vi "PIL_Main.vi"() -> ()   [LabVIEW 2024]
uses:
  controls/EXPERIMENT_Inputs.ctl
  controls/LASER_Inputs.ctl
  controls/LAMP_Inputs.ctl
  controls/GAS_Inputs.ctl
  controls/EXPERT_Inputs.ctl
  controls/XML_Inputs.ctl
  controls/SOFTWARE_Inputs.ctl
  controls/HSDIO_6541_Inputs.ctl
  <instrlib>/niHSDIO/niHSDIO.llb/niHSDIO_ctl Trigger Source Values (Ring).ctl
  controls/AWG_5421_Inputs.ctl
  <instrlib>/niFgen/niFgen.llb/niFgen_ctl Trigger Source Values (Ring).ctl
  controls/DIGIT_5122_Inputs.ctl
  <instrlib>/niScope/Controls/niScope trigger source.ctl
  controls/AO_6711_Inputs.ctl
  controls/AO_6738_Inputs.ctl
  controls/VOLTAGES_Inputs.ctl
  controls/HEXA_Inputs.ctl
  controls/QUAD_Inputs.ctl
  controls/SEQUENCE_Inputs.ctl
  controls/EXCIT_Inputs.ctl
  controls/DATA_Inputs.ctl
  controls/TIMING_Inputs.ctl
  controls/PROCESSING_Inputs.ctl
  controls/TRAPPING_Inputs.ctl
  controls/RF_TRAPPING_Inputs.ctl
  controls/SPECTRUM.ctl
  controls/EXCIT_Table.ctl
  controls/TIMING_Table.ctl
  controls/TIMING_Mandatory_Items.ctl
  controls/TIMING_Optional_Items.ctl
  controls/PIL_Status.ctl
  controls/LOOPS_Inputs.ctl
  controls/OPO_Inputs.ctl
  controls/QMH_UI_Cluster.ctl
  controls/QMH_UI_References.ctl
  controls/QMH_UI_Report.ctl
  controls/QMH_UI_Command.ctl
  controls/QMH_ICR_Command.ctl
  controls/QMH_Status.ctl
  controls/EXPERT_Path_Selector.ctl
  <vilib>/Utility/error.llb/DialogType.ctl
  Global_Variables.vi
panel:
  in  "Save As":bool
  in  "error in (no error)":errorcluster
  in  "Start":bool
  in  "Load":bool
  in  "Exit":bool
  in  "Tabs":T1(tab)=enum."Sequence"
  out "SPECTRUM":T2={"Day Path"=path "D:/PIRENEA/DATA/2016/data_2016_01_01", "Spectrum Name"="2016_01_01_000.A00", "Accumulated"=FALSE, "Stored in Database"=FALSE, "From a Set of"=0, "Quality Flag"="Optimal"}
  in  "Change Experiment":bool
  out "EXPERIMENT Inputs":T3={"Setup"="", "Date"="", "User Name"="", "Comment"="", "Experiment Procedures"=[], "Chemical Source"="", "Sample Components"=[], "Species"=[], "Laser 1"={"Used"=TRUE, "Name"="Spectroscopy", "Wavelength"=1000.0, "Energy"=25.0}, "Laser 2"={"Used"=TRUE, "Name"="Spectroscopy", "Wavelength"=1000.0, "Energy"=25.0}, "Laser 3"={"Used"=TRUE, "Name"="Spectroscopy", "Wavelength"=1000.0, "Energy"=25.0}, "Laser 4"={"Used"=TRUE, "Name"="Spectroscopy", "Wavelength"=1000.0, "Energy"=25.0}, "Laser 5"={"Used"=TRUE, "Name"="Spectroscopy", "Wavelength"=1000.0, "Energy"=25.0}, "Lamp 1"={"Used"=TRUE, "Name"="Spectroscopy", "Wavelength"=1000.0, "Attenuation"=25.0}, "Lamp 2"={"Used"=TRUE, "Name"="Spectroscopy", "Wavelength"=1000.0, "Attenuation"=25.0}, "Gas 1"={"Used"=TRUE, "Name"="Spectroscopy", "Pressure"=1000.0}, "Gas 2"={"Used"=TRUE, "Name"="Spectroscopy", "Pressure"=1000.0}, "Gas 3"={"Used"=TRUE, "Name"="Spectroscopy", "Pressure"=1000.0}, "Gas 4"={"Used"=TRUE, "Name"="Spectroscopy", "Pressure"=1000.0}, "Gas 5"={"Used"=TRUE, "Name"="Spectroscopy", "Pressure"=1000.0}} caption="EXCIT Paths"
  in  "Change Voltages":bool
  out "VOLTAGES Inputs":T7={"Hexa 1"={"Used"=FALSE, "Voltage"=0.0}, "Hexa 2"={"Used"=FALSE, "Voltage"=0.0}, "Hexa 3"={"Used"=FALSE, "Voltage"=0.0}, "Quad 1"={"Used"=TRUE, "Voltage"=25.0}, "Quad 2"={"Used"=TRUE, "Voltage"=25.0}, "Quad 3"={"Used"=TRUE, "Voltage"=25.0}}
  out "SEQUENCE Inputs":T10={"EXCIT Inputs"={"Number of Excitations"=1, "Script Text"="script  excit1wfm\r    wait until scriptTrigger0\r    generate Sinus250to500a25dur1200fs10\rend script", "Table of Waveforms"=["Sinus250to500a25dur1200fs10"]}, "DATA Inputs"={"Record Length"=524000, "Sample Rate"=2000000.0, "Data Type"=0, "Vertical Range"=2.0, "Acquisition Duration"=100000.0}, "TIMING Inputs"={"Number of Acquisitions "=1, "Number of Accumulations"=1, "Table of Waveforms"=["", "", "", "", "", "", "", "", "", "", "", ""], "Script Text"=""}, "PROCESSING Inputs"={"Reference Mass"=300.0939, "Cyclotron Freq"=255.727, "Magnetron Freq"=0.001}, "TRAPPING Inputs"={"Number of Channels"=4, "Init Values"=[2.0, 9.0, 9.0, 2.0], "Opening Values"=[0.0, 0.0, 0.0, 0.0], "Trapping Values"=[2.0, 9.0, 9.0, 2.0], "Emptying Values"=[-10.0, -10.0, -10.0, -10.0], "Adiabatic ON"=FALSE, "Adiabatic Duration"=0, "Adiabatic Waveforms"=["Adiabatic_None_2_2_2000", "Adiabatic_Ramp_9_0_2000", "Adiabatic_DoubleRamp_9_0_2000", "Adiabatic_RC_2_0_2000.bin"], "Ions Refill ON"=FALSE, "Number of Ions Refills"=4}, "RF_TRAPPING Inputs"={"Init Values"=[0.0, 1.0, 1.0, 0.0], "Opening Values"=[0.0, -4.0, 1.0, 0.0], "Trapping Values"=[0.0, 1.0, 1.0, 0.0], "Emptying Values"=[0.0, 1.0, -7.0, 0.0], "RF Trap ON"=FALSE, "RF Accums"=1, "Number of Voltages"=4}} {"RF_TRAPPING Inputs"."RF Accums" min=1 max=100; "RF_TRAPPING Inputs"."Trapping Values" min=-10.0 max=10.0; "RF_TRAPPING Inputs"."Init Values" min=-10.0 max=10.0; "RF_TRAPPING Inputs"."Emptying Values" min=-10.0 max=10.0; "RF_TRAPPING Inputs"."Opening Values" min=-10.0 max=10.0; "TRAPPING Inputs"."Number of Ions Refills" min=1 max=1000; "TRAPPING Inputs"."Trapping Values" min=-10.0 max=10.0; "TRAPPING Inputs"."Init Values" min=-10.0 max=10.0; "TRAPPING Inputs"."Emptying Values" min=-10.0 max=10.0; "TRAPPING Inputs"."Opening Values" min=-10.0 max=10.0; "PROCESSING Inputs"."Magnetron Freq" format="%.5g"; "PROCESSING Inputs"."Cyclotron Freq" format="%.5g"; "PROCESSING Inputs"."Reference Mass" format="%.5g"; "TIMING Inputs"."Number of Accumulations" min=0 max=50 step=1; "TIMING Inputs"."Number of Acquisitions" min=1 max=10 step=1; "DATA Inputs"."Vertical Range" items=["0.2"=0.2, "0.4"=0.4, "1"=1.0, "2"=2.0, "4"=4.0, "10"=10.0]; "DATA Inputs"."Data Type" items=["I16", "DBL"]; "DATA Inputs"."Sample Rate" items=["1 MHz"=1000000.0, "2 MHz"=2000000.0, "5 MHz"=5000000.0, "10 MHz"=10000000.0, "20 MHz"=20000000.0, "25 MHz"=25000000.0, "50 MHz"=50000000.0, "100 MHz"=100000000.0]; "EXCIT Inputs"."Number of Excitations" min=1 max=10}
  in  "Change Sequence":bool
  in  "Change Expert":bool
  out "EXPERT Inputs":T17={"XML Inputs"={"Version Tag Name"="XML_Version", "Version String"="1.1"}, "SOFTWARE Inputs"={"Application Directory"=path "D:/S.O.F.T.S/LABVIEW/PIL", "Software Version"="17.0f2", "Data Path"=path "D:/PIRENEA/DATA", "XML Path"=path "D:/PIRENEA/DATA", "XML File Filter"="*.xml", "XML Saved Path"=path "D:/PIRENEA/SAVED_XML", "Excit Scripts Path"=path "D:/PIRENEA/TECHNICAL/EXCIT_SCRIPTS", "Excit Scripts File Filter"="*.txt", "Excit Waveforms Path"=path "D:/PIRENEA/TECHNICAL/EXCIT_WFMS", "Excit Waveforms File Filter"="*.bin", "Timing Scripts Path"=path "D:/PIRENEA/TECHNICAL/TIMING_SCRIPTS", "Timing Scripts File Filter"="*.txt", "Timing Waveforms Path"=path "D:/PIRENEA/TECHNICAL/TIMING_WFMS", "Timing Waveforms File Filter"="*.bin", "Trapping Waveforms Path"=path "D:/PIRENEA/TECHNICAL/TRAPPING_WFMS", "Trapping Waveforms File Filter"="*.bin"}, "HSDIO 6541 Inputs"={"Resource Name"="HSDIO_6541", "Clock Rate"=1000000.0, "Trigger Source"="PFI0"}, "AWG 5421 Inputs"={"Resource Name"="AWG_5421", "Sample Rate"=10000000.0, "Trigger Type"=2, "Trigger Source"="PFI0", "Waveform Gain"=0.31, "Digital Filter ON"=TRUE}, "DIGIT 5122 Inputs"={"Sample Rate"=5000000.0, "Resource Name"="DIGIT_5122", "Channel Name"="0", "Trigger Source"="VAL_EXTERNAL", "Vertical Range"=2.0, "Trigger Level"=3.0}, "AO 6711 Inputs"={"Physical Channels"="AO_6711/ao0:3", "Min Voltage"=-10.0, "Max Voltage"=10.0, "Trigger Source"="/AO_6711/PFI3", "Counter"="AO_6711/ctr0"}, "AO 6738 Inputs"={"Physical Channels"="AO_6738/ao0:3", "Min Voltage"=-10.0, "Max Voltage"=10.0, "Trigger Source"="/AO_6738/PFI2", "Counter"="AO_6738/ctr0"}} {"AO 6738 Inputs"."Max Voltage" min=-10.0 max=10.0; "AO 6738 Inputs"."Min Voltage" min=-10.0 max=10.0; "AWG 5421 Inputs"."Sample Rate" format="%.2p"; "AWG 5421 Inputs"."Trigger Type" items=["None", "Software Edge", "Digital Edge", "Digital Level"]; "AO 6711 Inputs"."Max Voltage" min=-10.0 max=10.0; "AO 6711 Inputs"."Min Voltage" min=-10.0 max=10.0; "HSDIO 6541 Inputs"."Clock Rate" format="%.2p"; "DIGIT 5122 Inputs"."Trigger Level" format="%.2f"; "DIGIT 5122 Inputs"."Vertical Range" format="%.2f"; "DIGIT 5122 Inputs"."Sample Rate" step=65535.0 format="%#_3p"}
  in  "LOOPS Inputs":T28={"Number of Loops"=0, "Loop Current Value"=0, "OPO Inputs"={"OPO AutoAlignment ON"=FALSE, "OPO Start Value"=210.0, "OPO Stop Value"=270.0, "OPO Step"=30.0}} {"OPO Inputs"."OPO Step" min=0.5 max=60.0 format="%#.1f"; "OPO Inputs"."OPO Stop Value" min=210.0 max=270.0 format="%#.1f"; "OPO Inputs"."OPO Start Value" min=210.0 max=270.0 format="%#.1f"}
  in  "Change Loops":bool
  in  "Excit Test":bool caption="AWG5421 Board"
  out "TIMING Script":string
  in  "Change Scientist":bool
  out "TIMING Table":T30={"Mandatory Items"={"Script Name"="", "GINI Time Period"=100.0, "HSDIO Delay"=60.0, "Shutter Duration before"=50.0, "Shutter Duration after"=50.0, "Filter Tau"=2.0, "Trapping Delay"=600.0, "Trapping Duration"=300.0, "Emtyping Duration"=1000.0}, "Optional Items"={"Eject"=0, "Acq"=0, "Excit"=0, "Gas"=0, "Laser"=0, "Lamp"=0}, "Times Table"=[["Excit1", "name", "Swift", "0.5", "1200", "70", "150", "550", "0", "0", "0"]]} {"Optional Items"."Laser" min=0 max=3; "Optional Items"."Gas" min=0 max=5; "Mandatory Items"."GINI Time Period" min=100000.0 max=1000000.0 format="%#_7g"; "Mandatory Items"."Shutter Duration after" min=2.0 max=100000.0; "Mandatory Items"."HSDIO Delay" min=60.0 max=100.0; "Mandatory Items"."Shutter Duration before" min=2.0 max=100000.0; "Mandatory Items"."Filter Tau" min=1000.0 max=2000.0; "Mandatory Items"."Trapping Delay" min=2.0; "Mandatory Items"."Emtyping Duration" min=2.0 format="%#_8g"; "Mandatory Items"."Trapping Duration" min=2.0}
  out "EXCIT Table":T33={"Number of Excits"=0, "Number of Ejects"=0, "Sampling Frequency"=0.0, "Waveforms Table"=[["Excit1", "name", "Swift", "0.5", "1200", "70", "150", "550", "0", "0", "0"]]}
  out "PIL Status":T34
  # "Lasers"
  # "nm"
  # "mJ"
  # "Lamps"
  # "nm"
  # "dB"
  # "Gas"
  # "bar"
  # "HEXAPOLE"
  # "QUADRIPOLE"
  # "RF_V1"
  # "RF_V2"
  # "RF_V3"
  # "RF_V4"
  # "GO_out"
  # "Gout"
  # "GI_in"
  # "Gin"
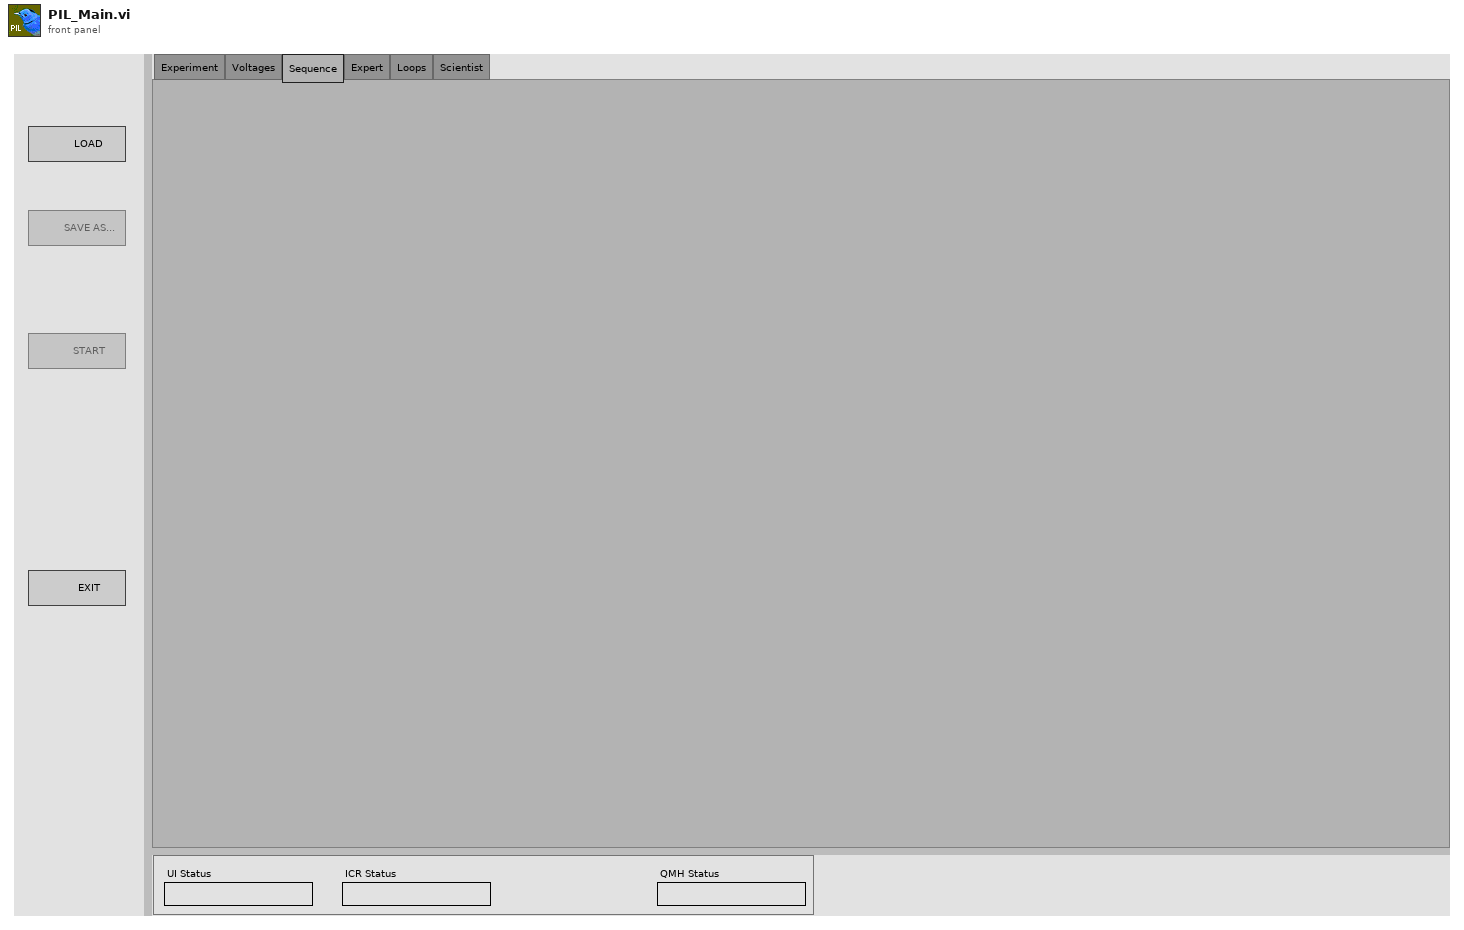
[diagram p1: front panel]
types:
  T1 = enum32{"Experiment", "Voltages", "Sequence", "Expert", "Loops", "Scientist"}
  T2 = typedef "SPECTRUM.ctl" = cluster{"Day Path":path, "Spectrum Name":string, "Accumulated":bool, "Stored in Database":bool, "From a Set of":i16, "Quality Flag":string}
  T3 = typedef "EXPERIMENT_Inputs.ctl" = cluster{"Setup":string, "Date":string, "User Name":string, "Comment":string, "Experiment Procedures":string[], "Chemical Source":string, "Sample Components":string[], "Species":string[], "Laser 1":T4, "Laser 2":T4, "Laser 3":T4, "Laser 4":T4, "Laser 5":T4, "Lamp 1":T5, "Lamp 2":T5, "Gas 1":T6, "Gas 2":T6, "Gas 3":T6, "Gas 4":T6, "Gas 5":T6}
  T4 = typedef "LASER_Inputs.ctl" = cluster{"Used":bool, "Name":string, "Wavelength":dbl, "Energy":dbl}
  T5 = typedef "LAMP_Inputs.ctl" = cluster{"Used":bool, "Name":string, "Wavelength":dbl, "Attenuation":dbl}
  T6 = typedef "GAS_Inputs.ctl" = cluster{"Used":bool, "Name":string, "Pressure":dbl}
  T7 = typedef "VOLTAGES_Inputs.ctl" = cluster{"Hexa 1":T8, "Hexa 2":T8, "Hexa 3":T8, "Quad 1":T9, "Quad 2":T9, "Quad 3":T9}
  T8 = typedef "HEXA_Inputs.ctl" = cluster{"Used":bool, "Voltage":dbl}
  T9 = typedef "QUAD_Inputs.ctl" = cluster{"Used":bool, "Voltage":dbl}
  T10 = typedef "SEQUENCE_Inputs.ctl" = cluster{"EXCIT Inputs":T11, "DATA Inputs":T12, "TIMING Inputs":T13, "PROCESSING Inputs":T14, "TRAPPING Inputs":T15, "RF_TRAPPING Inputs":T16}
  T11 = typedef "EXCIT_Inputs.ctl" = cluster{"Number of Excitations":i32, "Script Text":string, "Table of Waveforms":string[]}
  T12 = typedef "DATA_Inputs.ctl" = cluster{"Record Length":i32, "Sample Rate":dbl, "Data Type":u8, "Vertical Range":dbl, "Acquisition Duration":dbl}
  T13 = typedef "TIMING_Inputs.ctl" = cluster{"Number of Acquisitions ":i16, "Number of Accumulations":i16, "Table of Waveforms":string[], "Script Text":string}
  T14 = typedef "PROCESSING_Inputs.ctl" = cluster{"Reference Mass":dbl, "Cyclotron Freq":dbl, "Magnetron Freq":dbl}
  T15 = typedef "TRAPPING_Inputs.ctl" = cluster{"Number of Channels":i32, "Init Values":dbl[], "Opening Values":dbl[], "Trapping Values":dbl[], "Emptying Values":dbl[], "Adiabatic ON":bool, "Adiabatic Duration":i32, "Adiabatic Waveforms":string[], "Ions Refill ON":bool, "Number of Ions Refills":i32}
  T16 = typedef "RF_TRAPPING_Inputs.ctl" = cluster{"Init Values":dbl[], "Opening Values":dbl[], "Trapping Values":dbl[], "Emptying Values":dbl[], "RF Trap ON":bool, "RF Accums":i32, "Number of Voltages":i32}
  T17 = typedef "EXPERT_Inputs.ctl" = cluster{"XML Inputs":T18, "SOFTWARE Inputs":T19, "HSDIO 6541 Inputs":T20, "AWG 5421 Inputs":T22, "DIGIT 5122 Inputs":T24, "AO 6711 Inputs":T26, "AO 6738 Inputs":T27}
  T18 = typedef "XML_Inputs.ctl" = cluster{"Version Tag Name":string, "Version String":string}
  T19 = typedef "SOFTWARE_Inputs.ctl" = cluster{"Application Directory":path, "Software Version":string, "Data Path":path, "XML Path":path, "XML File Filter":string, "XML Saved Path":path, "Excit Scripts Path":path, "Excit Scripts File Filter":string, "Excit Waveforms Path":path, "Excit Waveforms File Filter":string, "Timing Scripts Path":path, "Timing Scripts File Filter":string, "Timing Waveforms Path":path, "Timing Waveforms File Filter":string, "Trapping Waveforms Path":path, "Trapping Waveforms File Filter":string}
  T20 = typedef "HSDIO_6541_Inputs.ctl" = cluster{"Resource Name":refnum<k15>, "Clock Rate":dbl, "Trigger Source":T21}
  T21 = typedef "niHSDIO_ctl Trigger Source Values (Ring).ctl" = string
  T22 = typedef "AWG_5421_Inputs.ctl" = cluster{"Resource Name":refnum<k15>, "Sample Rate":dbl, "Trigger Type":u16, "Trigger Source":T23, "Waveform Gain":dbl, "Digital Filter ON":bool}
  T23 = typedef "niFgen_ctl Trigger Source Values (Ring).ctl" = string
  T24 = typedef "DIGIT_5122_Inputs.ctl" = cluster{"Sample Rate":dbl, "Resource Name":refnum<k15>, "Channel Name":string, "Trigger Source":T25, "Vertical Range":dbl, "Trigger Level":dbl}
  T25 = typedef "niScope trigger source.ctl" = string
  T26 = typedef "AO_6711_Inputs.ctl" = cluster{"Physical Channels":tag, "Min Voltage":dbl, "Max Voltage":dbl, "Trigger Source":tag, "Counter":tag}
  T27 = typedef "AO_6738_Inputs.ctl" = cluster{"Physical Channels":tag, "Min Voltage":dbl, "Max Voltage":dbl, "Trigger Source":tag, "Counter":tag}
  T28 = typedef "LOOPS_Inputs.ctl" = cluster{"Number of Loops":i16, "Loop Current Value":i16, "OPO Inputs":T29}
  T29 = typedef "OPO_Inputs.ctl" = cluster{"OPO AutoAlignment ON":bool, "OPO Start Value":dbl, "OPO Stop Value":dbl, "OPO Step":dbl}
  T30 = typedef "TIMING_Table.ctl" = cluster{"Mandatory Items":T31, "Optional Items":T32, "Times Table":string[][]}
  T31 = typedef "TIMING_Mandatory_Items.ctl" = cluster{"Script Name":string, "GINI Time Period":dbl, "HSDIO Delay":dbl, "Shutter Duration before":dbl, "Shutter Duration after":dbl, "Filter Tau":dbl, "Trapping Delay":dbl, "Trapping Duration":dbl, "Emtyping Duration":dbl}
  T32 = typedef "TIMING_Optional_Items.ctl" = cluster{"Eject":u32, "Acq":i32, "Excit":u32, "Gas":i32, "Laser":i32, "Lamp":i32}
  T33 = typedef "EXCIT_Table.ctl" = cluster{"Number of Excits":u16, "Number of Ejects":u16, "Sampling Frequency":dbl, "Waveforms Table":string[][]}
  T34 = typedef "PIL_Status.ctl" = cluster{"UI Status":string, "ICR Status":string, "QMH Status":string}
  T35 = typedef "QMH_UI_Cluster.ctl" = cluster{"QMH UI References":T36, "QMH UI Report":T37}
  T36 = typedef "QMH_UI_References.ctl" = cluster{"Refnum Load":refnum<vi>, "Refnum Save As":refnum<vi>, "Refnum Start":refnum<vi>, "Refnum Exit":refnum<vi>, "Refnum Tabs":refnum<vi>, "Refnum SPECTRUM":refnum<vi>, "Refnum EXPERIMENT":refnum<vi>, "Refnum VOLTAGES":refnum<vi>, "Refnum SEQUENCE":refnum<vi>, "Refnum EXPERT":refnum<vi>, "Refnum LOOPS":refnum<vi>, "Refnum EXCIT Table":refnum<vi>, "Refnum TIMING Table":refnum<vi>, "Refnum CHANGE Experiment":refnum<vi>, "Refnum CHANGE Voltages":refnum<vi>, "Refnum CHANGE Sequence":refnum<vi>, "Refnum CHANGE Expert":refnum<vi>, "Refnum CHANGE Loops":refnum<vi>, "Refnum CHANGE Scientist":refnum<vi>, "Refnum PIL Status":refnum<vi>}
  T37 = typedef "QMH_UI_Report.ctl" = cluster{"UI Status":T38, "ICR Status":T39, "QMH Status":T40}
  T38 = typedef "QMH_UI_Command.ctl" = enum16{"Initialize", "UI Load", "UI Save", "UI Save As", "UI Change Experiment", "UI Change Voltages", "UI Change Sequence", "UI Change Expert", "UI Change Loops", "UI Change Scientist", "Ready to Start", "UI Start", "Waiting for ICR", "UI Exit", "Update Experiment", "Update Report", "Update ICR Status", "Waiting for User"}
  T39 = typedef "QMH_ICR_Command.ctl" = enum16{"Initialize", "Sequence Loop Setup", "Sequence Setup", "ICR Start", "ICR Stop", "Hardware Setup", "Next Sequence Loop", "Next Accumulation", "Waiting for Trigger", "Sequence Started", "Sequence Finished", "Sequence Loop Done", "Writing Data", "Hardware Reset", "Exit"}
  T40 = typedef "QMH_Status.ctl" = enum16{"Init", "Loading", "Setup", "Ready to Start", "Started", "Idle"}
  T41 = typedef "EXPERT_Path_Selector.ctl" = enum16{"Application", "Resources", "Data", "XML", "XML Saved", "Load Directory"}
  T42 = typedef "QMH_UI_Message.ctl" = cluster{"Command":T38, "Data":variant}
  T43 = typedef "DialogType.ctl" = u16
  T44 = enum32{"invalid app kind", "Development System", "Run Time System", "Student Edition", "Embedded LabVIEW", "Evaluation", "Custom"}
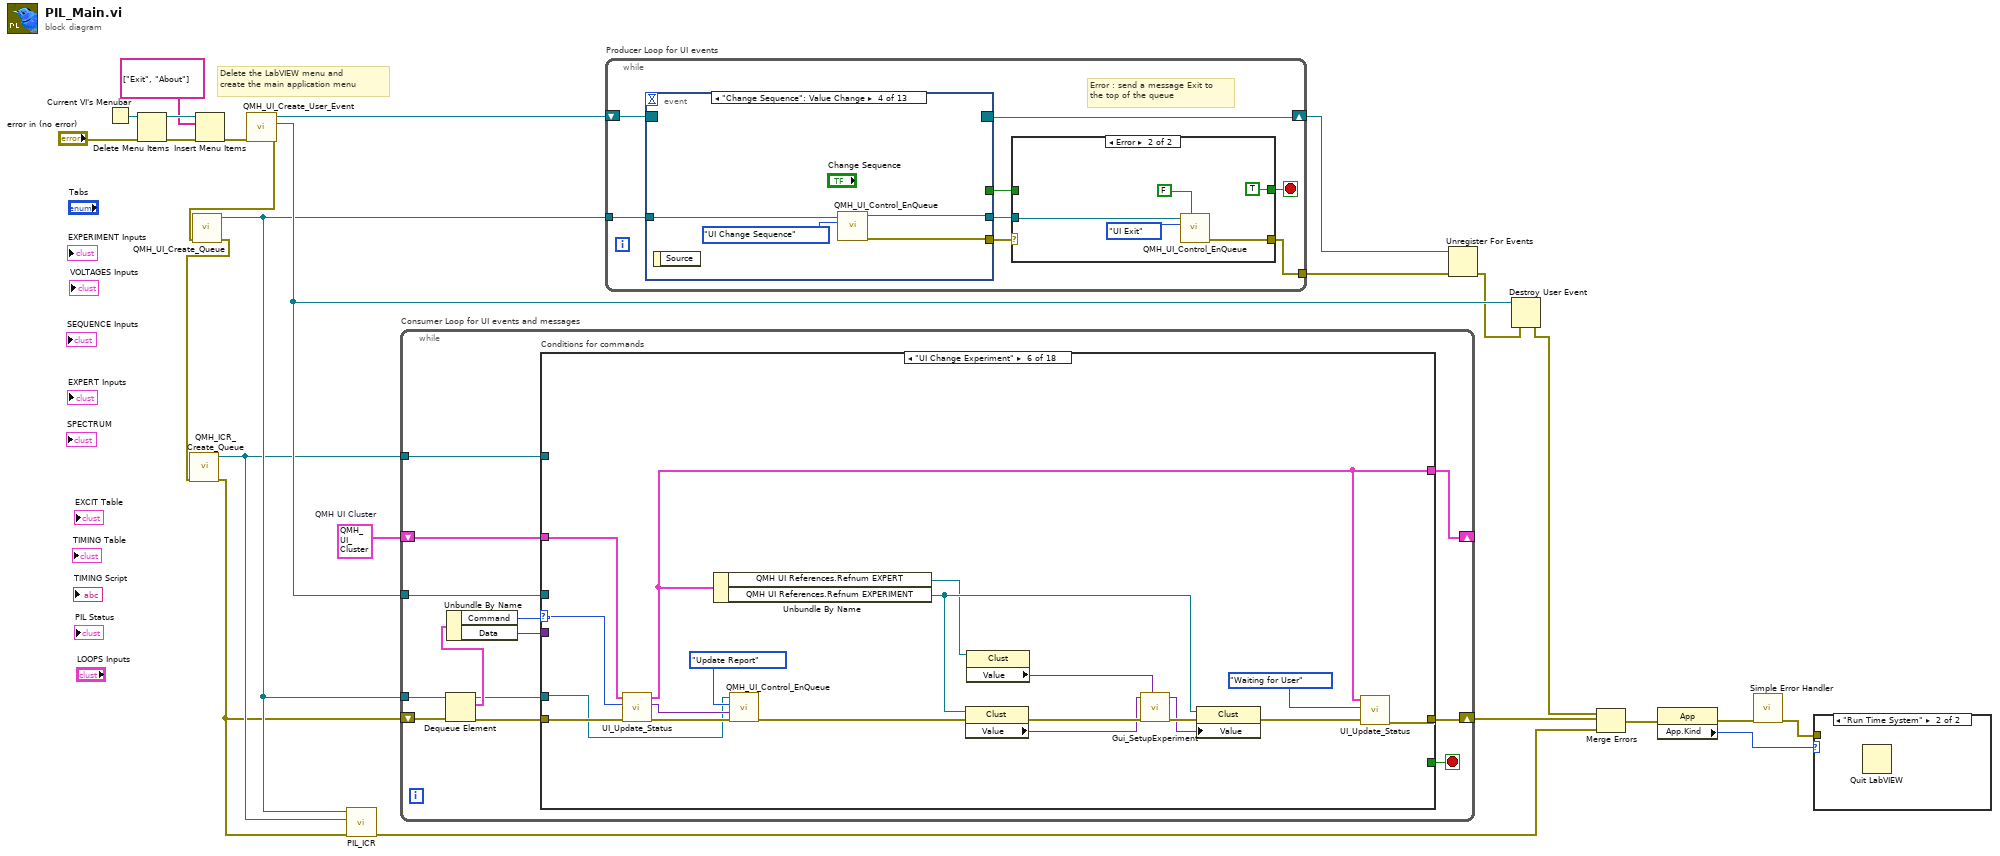
[diagram p0: block diagram]
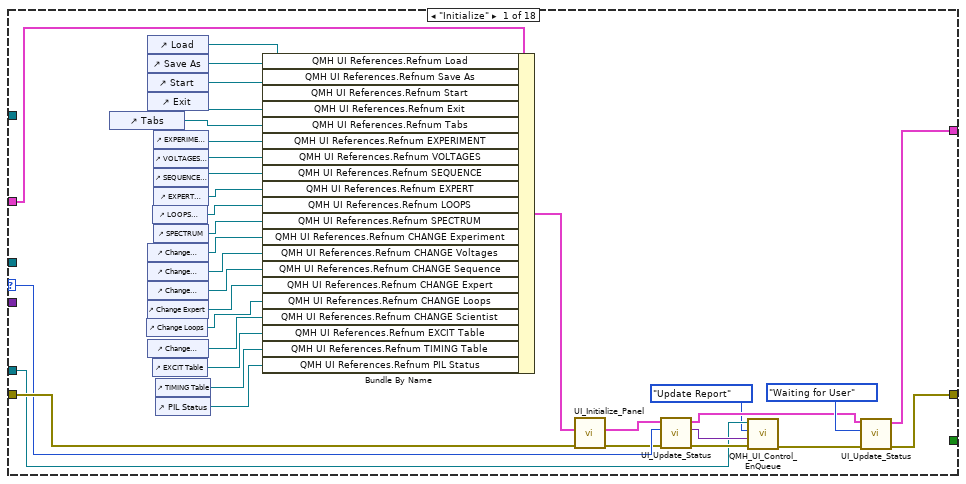
[diagram p2: hidden frame]
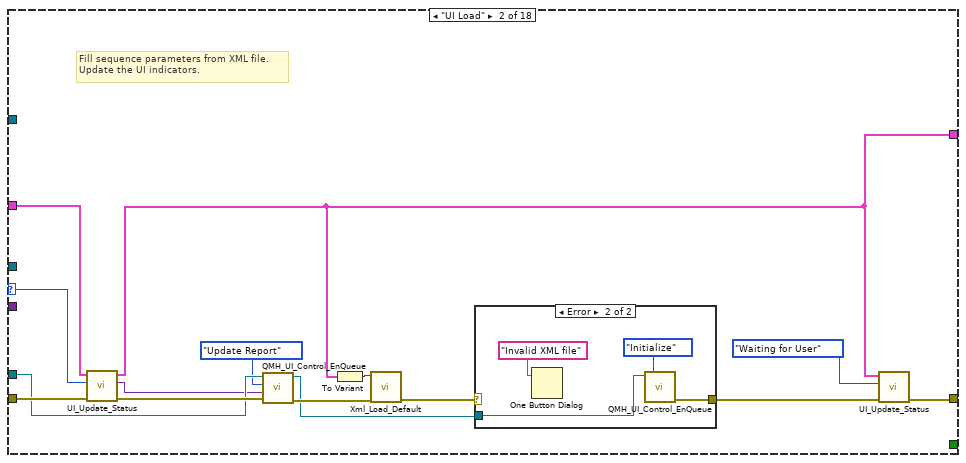
[diagram p3: hidden frame]
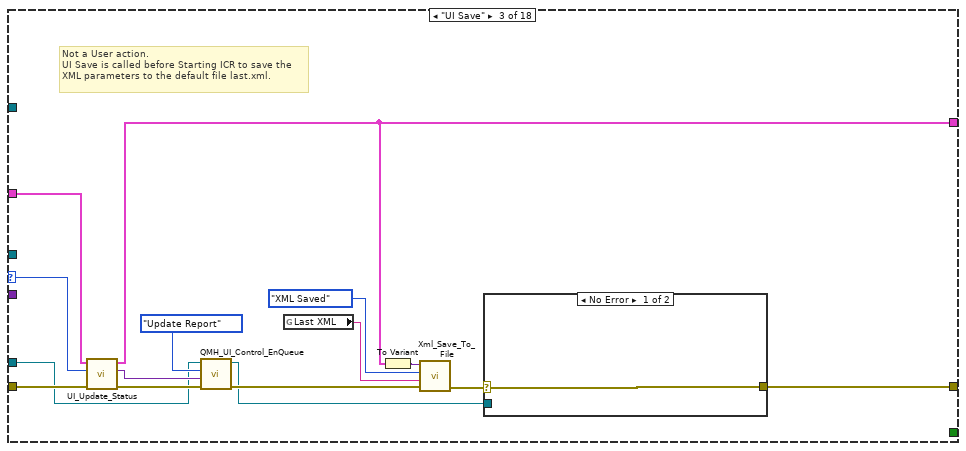
[diagram p5: hidden frame]
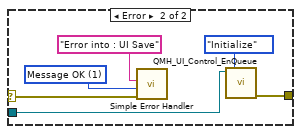
[diagram p6: hidden frame]
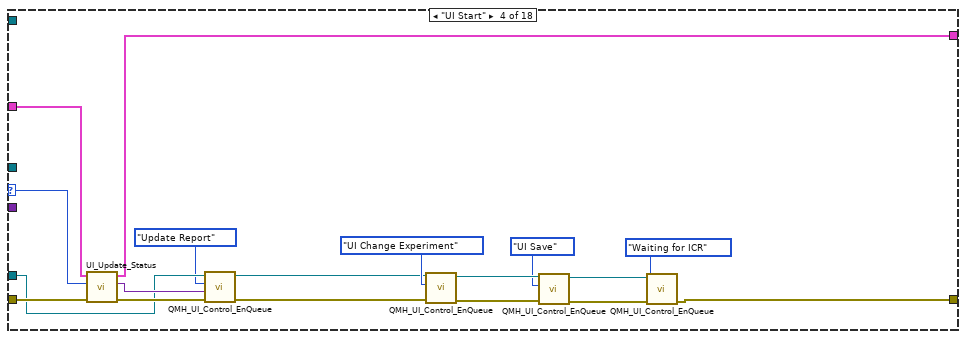
[diagram p7: hidden frame]
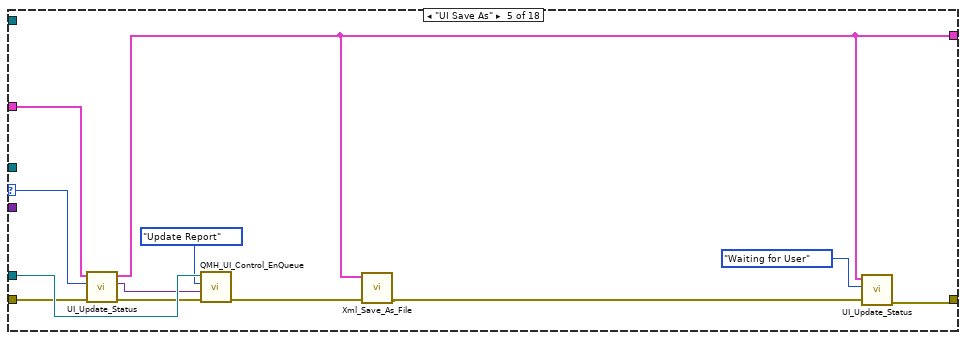
[diagram p8: hidden frame]
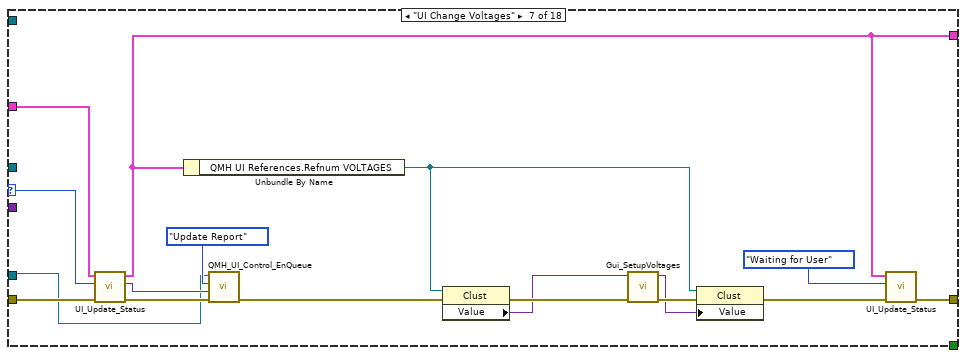
[diagram p9: hidden frame]
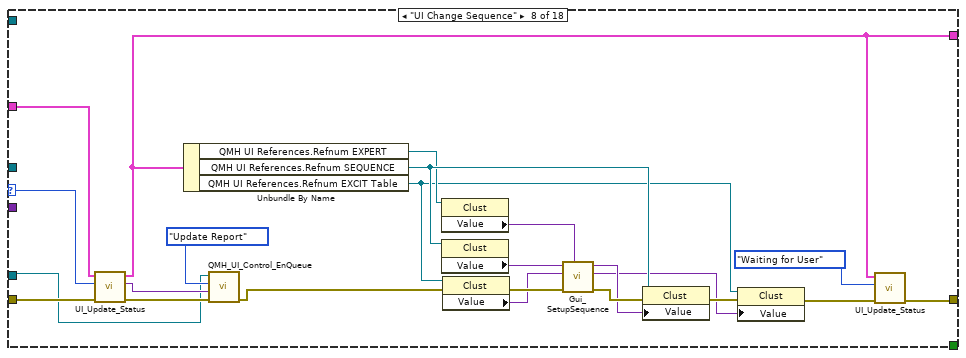
[diagram p10: hidden frame]
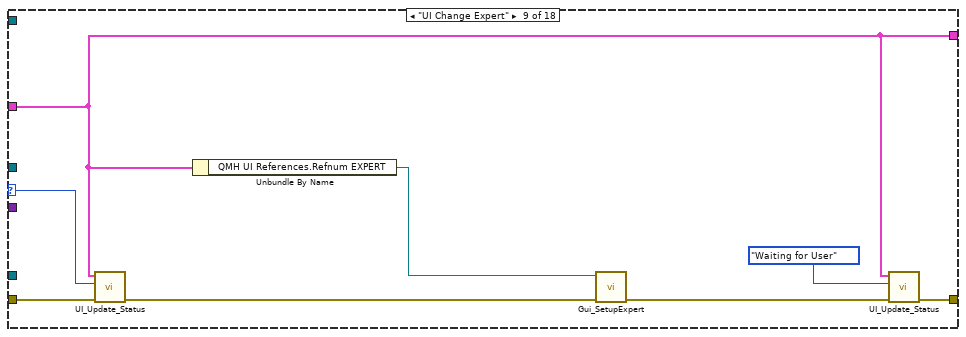
[diagram p11: hidden frame]
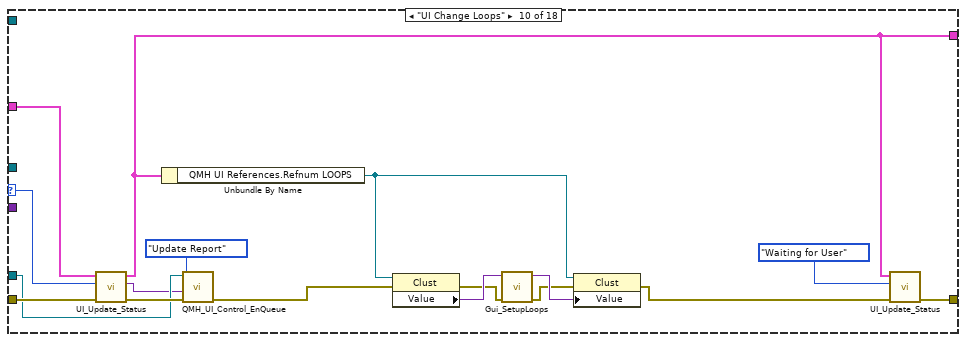
[diagram p12: hidden frame]
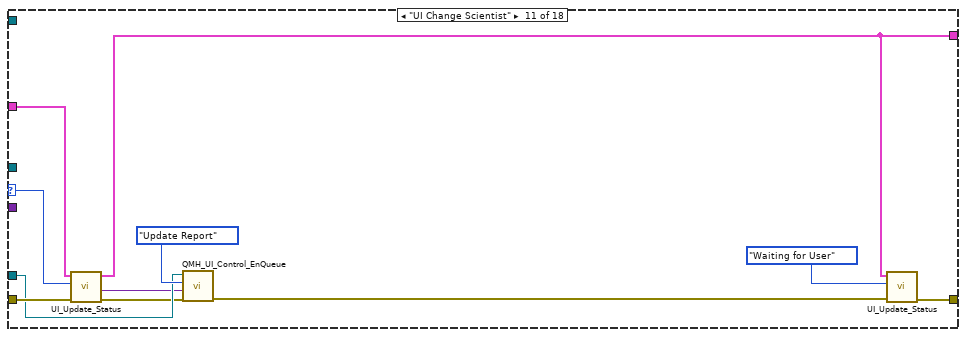
[diagram p13: hidden frame]
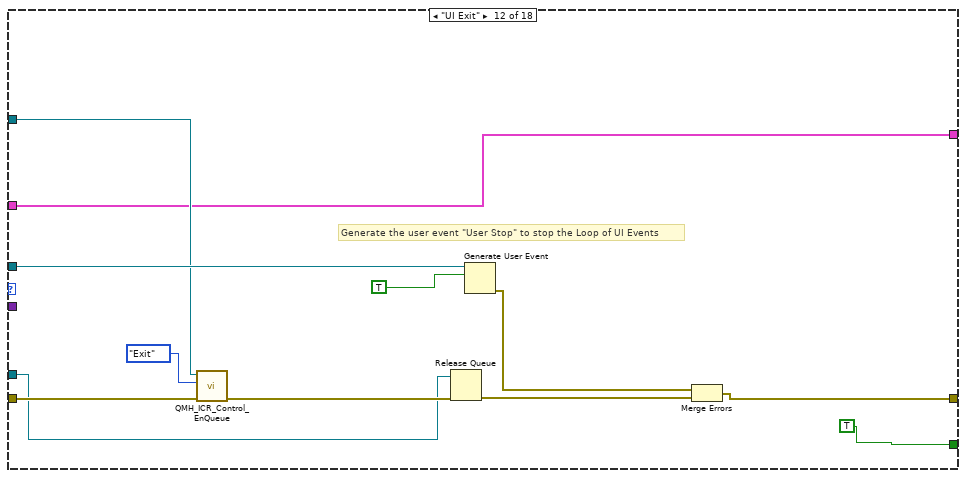
[diagram p14: hidden frame]
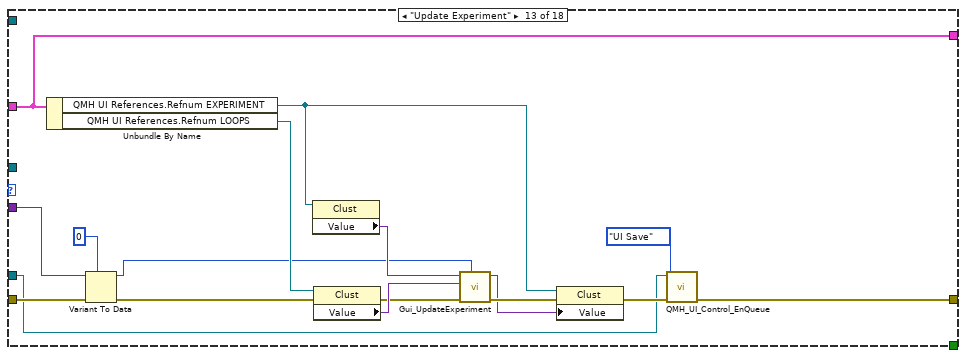
[diagram p15: hidden frame]
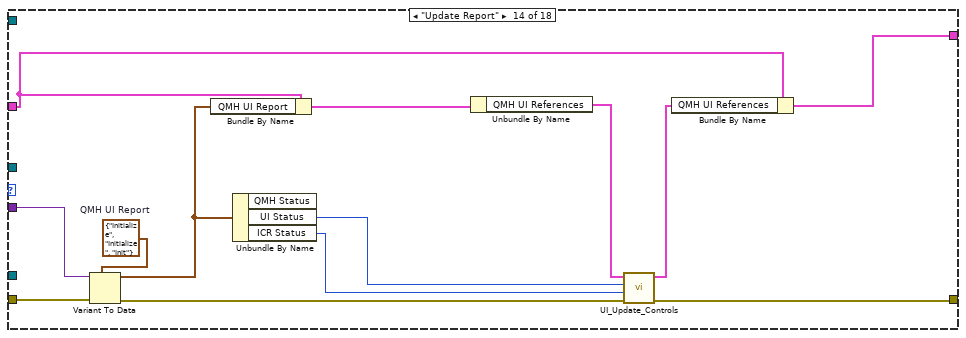
[diagram p16: hidden frame]
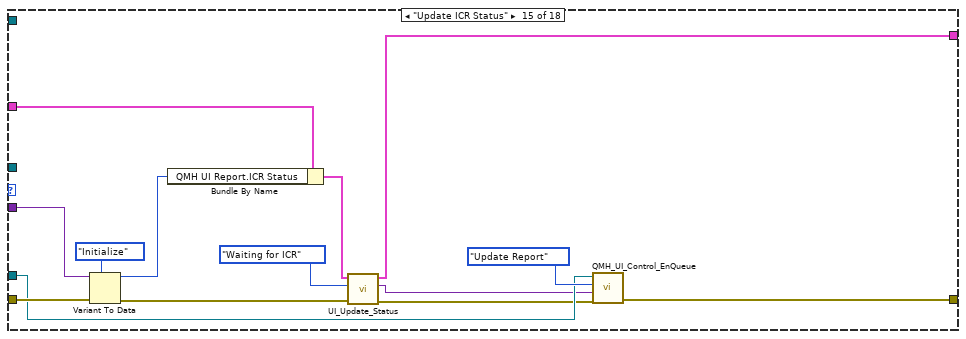
[diagram p17: hidden frame]
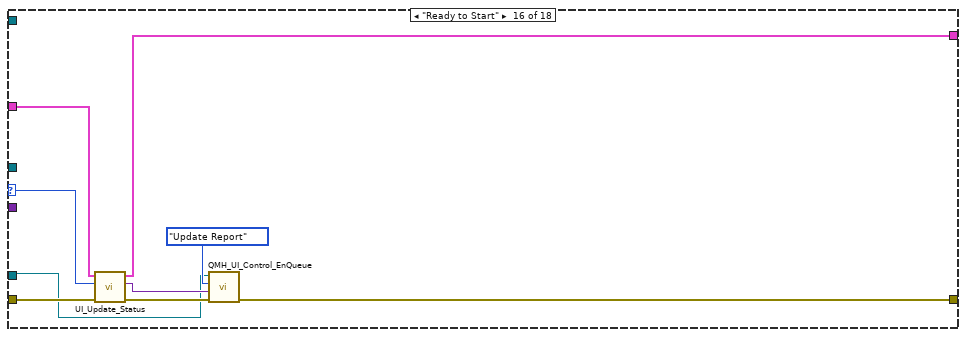
[diagram p18: hidden frame]
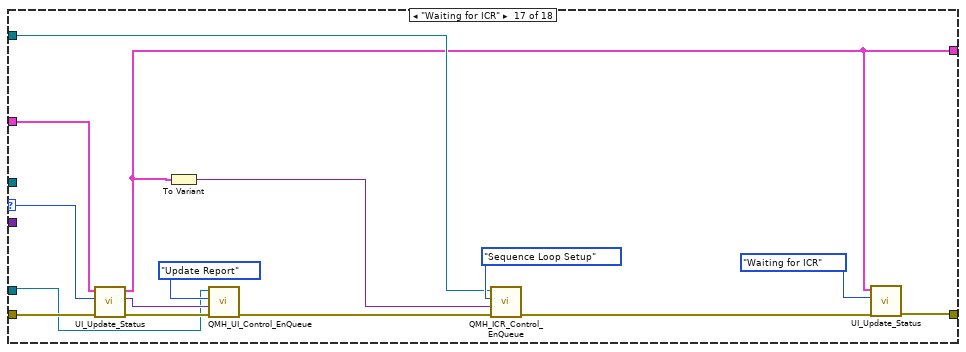
[diagram p19: hidden frame]
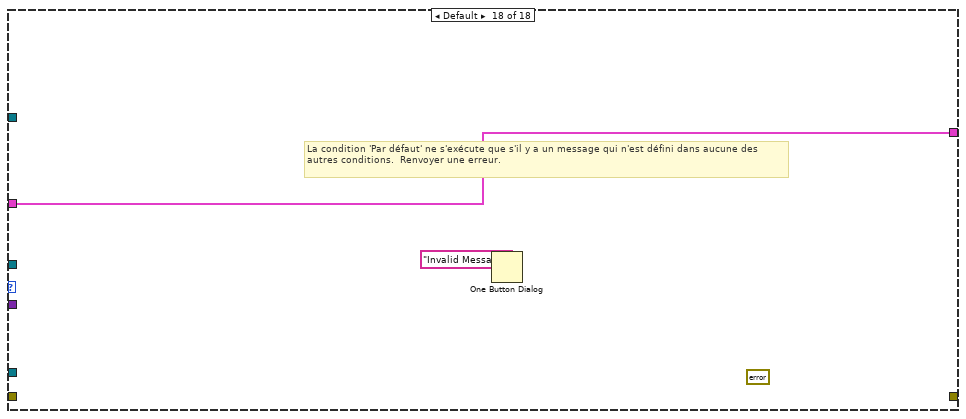
[diagram p20: hidden frame]
diagram:
  w23 = T35 {"QMH UI References"={"Refnum Load"=refnum, "Refnum Save As"=refnum, "Refnum Start"=refnum, "Refnum Exit"=refnum, "Refnum Tabs"=refnum, "Refnum SPECTRUM"=refnum, "Refnum EXPERIMENT"=refnum, "Refnum VOLTAGES"=refnum, "Refnum SEQUENCE"=refnum, "Refnum EXPERT"=refnum, "Refnum LOOPS"=refnum, "Refnum EXCIT Table"=refnum, "Refnum TIMING Table"=refnum, "Refnum CHANGE Experiment"=refnum, "Refnum CHANGE Voltages"=refnum, "Refnum CHANGE Sequence"=refnum, "Refnum CHANGE Expert"=refnum, "Refnum CHANGE Loops"=refnum, "Refnum CHANGE Scientist"=refnum, "Refnum PIL Status"=refnum}, "QMH UI Report"={"UI Status"=enum."Initialize", "ICR Status"=enum."Initialize", "QMH Status"=enum."Init"}}  # QMH UI Cluster
  # "Delete the LabVIEW menu and\ncreate the main application menu"
  n1 = Current VI's Menubar() -> (w6:refnum<k9>)
  n2 = Delete Menu Items(6:"error in (no error)", 9:w6) -> (0:w5:errorcluster, 3:w4:refnum<k9>)  [unwired: 2 in]
  n3 = Insert Menu Items(6:w5, 8:string[] ["Exit", "About"] ("noms des éléments"), 9:w4) -> (0:w2:errorcluster)  [unwired: 3 in, 2 out]
  n4 = call "QMH_UI_Create_User_Event.vi"("error in (no error)"=w2) -> ("error out"=w22:errorcluster, "User Stop Event"=w18:refnum<user-event>, "Refnum register for events"=w24:refnum<event-registration>)  [unwired: 8 in]
  n5 = call "QMH_UI_Create_Queue.vi"("error in (no error)"=w22) -> ("error out"=w8:errorcluster, "UI Queue"=w11:refnum<queue>)  [unwired: 9 in]
  n6 = call "QMH_ICR_Create_Queue.vi"("error in (no error)"=w8) -> ("error out"=w7:errorcluster, "ICR Queue"=w10:refnum<queue>)  [unwired: 9 in]
  n7 = call "PIL_ICR.vi"("error in (no error)"=w7, "ICR Queue"=w10, "UI Queue"=w11) -> ("error out"=w9:errorcluster)  [unwired: 8 in]
  n8 = while "Consumer Loop for UI events and messages" {
    shift-right: [w28] -> _
    shift-left: w23 -> [w37]
    shift-right: [w26] -> w19
    shift-left: w7 -> [w33]
    tunnel: w11 -> [w34]
    tunnel: w18 -> [w29]
    tunnel: w10 -> [w25]
    stop <- w36 stop-if-true
    n9 = Dequeue Element(queue=w34, error in (no error)=w33) -> (queue out=w32:refnum<queue>, element=w35:T42, error out=w27:errorcluster)  [unwired: 2 out]
    n10 = Unbundle By Name(w35) -> ("Command"=w31:T38, "Data"=w30:variant)
    n11 = case "Conditions for commands" shown="\"UI Change Experiment\"" w31 {
      selector: w31 -> [w52 w86 w104 w131 w140 w158 w175 w198 w210 w227 w238 _ _ _ _ w300 w315 _]
      tunnel: w32 -> [w41 w77 w97 w123 w144 w156 w173 w196 _ w222 w233 w242 w254 _ w288 w298 w313 _]
      tunnel: w37 -> [w70 w81 w103 w130 w139 w159 w176 w199 w204 w224 w235 w240 w266 w271 w293 w301 w316 w320]
      tunnel: [_ _ _ _ _ _ _ _ _ _ _ TRUE _ _ _ _ _ _] -> w36
      tunnel: w30 -> [_ _ _ _ _ _ _ _ _ _ _ _ w268 w281 w295 _ _ _]
      tunnel: w29 -> [_ _ _ _ _ _ _ _ _ _ _ w248 _ _ _ _ _ _]
      tunnel: [w48 w74 w93 w119 w133 w145 w164 w182 w204 w212 w229 w240 w266 w277 w285 w297 w305 w320] -> w28
      tunnel: w27 -> [w53 w87 w105 w132 w141 w157 w174 w197 w209 w226 w239 w244 w267 w276 w294 w299 w314 _]
      tunnel: [w51 w82 w98 w117 w135 w146 w165 w183 w205 w225 w237 w246 w255 w275 w289 w296 w306 _] -> w26
      tunnel: w25 -> [_ _ _ _ _ _ _ _ _ _ _ w241 _ _ _ _ w311 _]
      frame "Initialize" {
        n12 = control-ref of="Tabs"() -> (w69:refnum<vi>)
        n13 = control-ref of="Change Loops"() -> (w39:refnum<vi>)
        n14 = control-ref of="Load"() -> (w72:refnum<vi>)
        n15 = control-ref of="Save As"() -> (w59:refnum<vi>)
        n16 = control-ref of="Start"() -> (w60:refnum<vi>)
        n17 = control-ref of="Exit"() -> (w71:refnum<vi>)
        n18 = control-ref of="Change Experiment"() -> (w64:refnum<vi>)
        n19 = control-ref of="Change Voltages"() -> (w61:refnum<vi>)
        n20 = control-ref of="Change Sequence"() -> (w62:refnum<vi>)
        n21 = control-ref of="Change Expert"() -> (w63:refnum<vi>)
        n22 = control-ref of="Change Scientist"() -> (w56:refnum<vi>)
        n23 = control-ref of="LOOPS Inputs"() -> (w38:refnum<vi>)
        n24 = control-ref of="EXCIT Table"() -> (w55:refnum<vi>)
        n25 = control-ref of="EXPERIMENT Inputs"() -> (w68:refnum<vi>)
        n26 = control-ref of="VOLTAGES Inputs"() -> (w67:refnum<vi>)
        n27 = control-ref of="SEQUENCE Inputs"() -> (w66:refnum<vi>)
        n28 = control-ref of="EXPERT Inputs"() -> (w58:refnum<vi>)
        n29 = control-ref of="SPECTRUM"() -> (w65:refnum<vi>)
        n30 = control-ref of="TIMING Table"() -> (w57:refnum<vi>)
        n31 = control-ref of="PIL Status"() -> (w54:refnum<vi>)
        n32 = Bundle By Name(cluster=w70, "QMH UI References.Refnum Load"=w72, "QMH UI References.Refnum Save As"=w59, "QMH UI References.Refnum Start"=w60, "QMH UI References.Refnum Exit"=w71, "QMH UI References.Refnum Tabs"=w69, "QMH UI References.Refnum EXPERIMENT"=w68, "QMH UI References.Refnum VOLTAGES"=w67, "QMH UI References.Refnum SEQUENCE"=w66, "QMH UI References.Refnum EXPERT"=w58, "QMH UI References.Refnum LOOPS"=w38, "QMH UI References.Refnum SPECTRUM"=w65, "QMH UI References.Refnum CHANGE Experiment"=w64, "QMH UI References.Refnum CHANGE Voltages"=w61, "QMH UI References.Refnum CHANGE Sequence"=w62, "QMH UI References.Refnum CHANGE Expert"=w63, "QMH UI References.Refnum CHANGE Loops"=w39, "QMH UI References.Refnum CHANGE Scientist"=w56, "QMH UI References.Refnum EXCIT Table"=w55, "QMH UI References.Refnum TIMING Table"=w57, "QMH UI References.Refnum PIL Status"=w54) -> (w46:T35)
        n33 = call "UI_Initialize_Panel.vi"("error in (no error)"=w53, "QMH UI Cluster"=w46) -> ("error out"=w47:errorcluster, "QMH UI Cluster"=w45:T35)  [unwired: 8 in]
        n34 = call "UI_Update_Status.vi"("error in (no error)"=w47, "UI Status"=w52, "QMH UI Cluster"=w45) -> ("error out"=w44:errorcluster, "Variant"=w43:variant, "QMH UI Cluster"=w49:T35)  [unwired: 6 in]
        n35 = call "QMH_UI_Control_EnQueue.vi"("error in (no error)"=w44, "Variant"=w43, "Command"=QMH_UI_Command."Update Report", "UI Queue"=w41) -> ("error out"=w42:errorcluster)  [unwired: 6 in, 1 out]
        n36 = call "UI_Update_Status.vi"("error in (no error)"=w42, "UI Status"=QMH_UI_Command."Waiting for User", "QMH UI Cluster"=w49) -> ("error out"=w51:errorcluster, "QMH UI Cluster"=w48:T35)  [unwired: 6 in, 1 out]
      }
      frame "UI Load" {
        # "Fill sequence parameters from XML file.\nUpdate the UI indicators."
        n37 = call "UI_Update_Status.vi"("error in (no error)"=w87, "UI Status"=w86, "QMH UI Cluster"=w81) -> ("error out"=w79:errorcluster, "Variant"=w73:variant, "QMH UI Cluster"=w74:T35)  [unwired: 6 in]
        n38 = call "QMH_UI_Control_EnQueue.vi"("error in (no error)"=w79, "Variant"=w73, "Command"=QMH_UI_Command."Update Report", "UI Queue"=w77) -> ("error out"=w78:errorcluster, "UI Queue"=w76:refnum<queue>)  [unwired: 6 in]
        n39 = To Variant(anything=w74) -> (Variant=w85:variant)
        n40 = call "Xml_Load_Default.vi"("error in (no error)"=w78, "Variant"=w85) -> ("error out"=w83:errorcluster)  [unwired: 9 in]
        n41 = case shown="Error" w83 {
          selector: w83 -> [w88 _]
          tunnel: [w88 w92] -> w84
          tunnel: w76 -> [_ w89]
          frame No Error {
          }
          frame Error {
            n42 = One Button Dialog(message="Invalid XML file") -> ()  [unwired: 1 in, 1 out]
            n43 = call "QMH_UI_Control_EnQueue.vi"("Command"=QMH_UI_Command."Initialize", "UI Queue"=w89) -> ("error out"=w92:errorcluster)  [unwired: 8 in, 1 out]
          }
        }
        n44 = call "UI_Update_Status.vi"("error in (no error)"=w84, "UI Status"=QMH_UI_Command."Waiting for User", "QMH UI Cluster"=w74) -> ("error out"=w82:errorcluster)  [unwired: 6 in, 2 out]
      }
      frame "UI Save" {
        # "Not a User action.\nUI Save is called before Starting ICR to save the\nXML parameters to the default file last.xml."
        n45 = call "UI_Update_Status.vi"("error in (no error)"=w105, "UI Status"=w104, "QMH UI Cluster"=w103) -> ("error out"=w106:errorcluster, "Variant"=w102:variant, "QMH UI Cluster"=w93:T35)  [unwired: 6 in]
        n46 = call "QMH_UI_Control_EnQueue.vi"("error in (no error)"=w106, "Variant"=w102, "Command"=QMH_UI_Command."Update Report", "UI Queue"=w97) -> ("error out"=w101:errorcluster, "UI Queue"=w94:refnum<queue>)  [unwired: 6 in]
        n47 = global read "Global_Variables.vi" "Last XML"() -> (w95:string)
        n48 = To Variant(anything=w93) -> (Variant=w100:variant)
        n49 = call "Xml_Save_To_File.vi"("error in (no error)"=w101, "Filename"=w95, "EXPERT Path Selector"=EXPERT_Path_Selector."XML Saved", "Variant"=w100) -> ("error out"=w99:errorcluster)  [unwired: 7 in]
        n50 = case shown="No Error" w99 {
          selector: w99 -> [w108 w111]
          tunnel: [w108 w114] -> w98
          tunnel: w94 -> [_ w112]
          frame No Error {
          }
          frame Error {
            w109 = T43 1 items=["pas de dialogue", "Message OK", "Message continuer ou arrêter", "Message OK + mises en garde", "Arrêter/Continuer + mises en garde"] ("type of dialog (OK msg:1)")
            n51 = call <vilib>:"Simple Error Handler.vi"("error source (\" \")"="Error into : UI Save" ("error source (\" \")"), "type of dialog (OK msg:1)"=w109, "error in (no error)"=w111) -> ()  [unwired: 2 in, 5 out]
            n52 = call "QMH_UI_Control_EnQueue.vi"("Command"=QMH_UI_Command."Initialize", "UI Queue"=w112) -> ("error out"=w114:errorcluster)  [unwired: 8 in, 1 out]
          }
        }
      }
      frame "UI Start" {
        n53 = call "UI_Update_Status.vi"("error in (no error)"=w132, "UI Status"=w131, "QMH UI Cluster"=w130) -> ("error out"=w125:errorcluster, "Variant"=w124:variant, "QMH UI Cluster"=w119:T35)  [unwired: 6 in]
        n54 = call "QMH_UI_Control_EnQueue.vi"("error in (no error)"=w125, "Variant"=w124, "Command"=QMH_UI_Command."Update Report", "UI Queue"=w123) -> ("error out"=w116:errorcluster, "UI Queue"=w115:refnum<queue>)  [unwired: 6 in]
        n55 = call "QMH_UI_Control_EnQueue.vi"("error in (no error)"=w116, "Command"=QMH_UI_Command."UI Change Experiment", "UI Queue"=w115) -> ("error out"=w128:errorcluster, "UI Queue"=w127:refnum<queue>)  [unwired: 7 in]
        n56 = call "QMH_UI_Control_EnQueue.vi"("error in (no error)"=w128, "Command"=QMH_UI_Command."UI Save", "UI Queue"=w127) -> ("error out"=w118:errorcluster, "UI Queue"=w121:refnum<queue>)  [unwired: 7 in]
        n57 = call "QMH_UI_Control_EnQueue.vi"("error in (no error)"=w118, "Command"=QMH_UI_Command."Waiting for ICR", "UI Queue"=w121) -> ("error out"=w117:errorcluster)  [unwired: 7 in, 1 out]
      }
      frame "UI Save As" {
        n58 = call "UI_Update_Status.vi"("error in (no error)"=w141, "UI Status"=w140, "QMH UI Cluster"=w139) -> ("error out"=w142:errorcluster, "Variant"=w138:variant, "QMH UI Cluster"=w133:T35)  [unwired: 6 in]
        n59 = call "QMH_UI_Control_EnQueue.vi"("error in (no error)"=w142, "Variant"=w138, "Command"=QMH_UI_Command."Update Report", "UI Queue"=w144) -> ("error out"=w137:errorcluster)  [unwired: 6 in, 1 out]
        n60 = call "Xml_Save_As_File.vi"("error in (no error)"=w137, "QMH UI Cluster"=w133) -> ("error out"=w136:errorcluster)  [unwired: 9 in]
        n61 = call "UI_Update_Status.vi"("error in (no error)"=w136, "UI Status"=QMH_UI_Command."Waiting for User", "QMH UI Cluster"=w133) -> ("error out"=w135:errorcluster)  [unwired: 6 in, 2 out]
      }
      frame "UI Change Experiment" {
        n62 = call "UI_Update_Status.vi"("error in (no error)"=w157, "UI Status"=w158, "QMH UI Cluster"=w159) -> ("error out"=w161:errorcluster, "Variant"=w160:variant, "QMH UI Cluster"=w145:T35)  [unwired: 6 in]
        n63 = Unbundle By Name(w145) -> ("QMH UI References.Refnum EXPERT"=w150:refnum<vi>, "QMH UI References.Refnum EXPERIMENT"=w155:refnum<vi>)
        n64 = call "QMH_UI_Control_EnQueue.vi"("error in (no error)"=w161, "Variant"=w160, "Command"=QMH_UI_Command."Update Report", "UI Queue"=w156) -> ("error out"=w154:errorcluster)  [unwired: 6 in, 1 out]
        n65 = property class="Clust"(reference=w155, error in=w154) -> (error out=w153:errorcluster, "Value"=w152:variant)  [unwired: 1 out]
        n66 = property class="Clust"(reference=w150) -> ("Value"=w149:variant)  [unwired: 1 in, 2 out]
        n67 = call "Gui_SetupExperiment.vi"("Variant for Path"=w149, "error in (no error)"=w153, "Variant"=w152) -> ("error out"=w163:errorcluster, "Variant Output"=w151:variant)  [unwired: 7 in]
        n68 = property class="Clust"(reference=w155, error in=w163, "Value"=w151) -> (error out=w147:errorcluster)  [unwired: 1 out]
        n69 = call "UI_Update_Status.vi"("error in (no error)"=w147, "UI Status"=QMH_UI_Command."Waiting for User", "QMH UI Cluster"=w145) -> ("error out"=w146:errorcluster)  [unwired: 6 in, 2 out]
      }
      frame "UI Change Voltages" {
        n70 = call "UI_Update_Status.vi"("error in (no error)"=w174, "UI Status"=w175, "QMH UI Cluster"=w176) -> ("error out"=w178:errorcluster, "Variant"=w177:variant, "QMH UI Cluster"=w164:T35)  [unwired: 6 in]
        n71 = Unbundle By Name(w164) -> ("QMH UI References.Refnum VOLTAGES"=w172:refnum<vi>)
        n72 = call "QMH_UI_Control_EnQueue.vi"("error in (no error)"=w178, "Variant"=w177, "Command"=QMH_UI_Command."Update Report", "UI Queue"=w173) -> ("error out"=w171:errorcluster)  [unwired: 6 in, 1 out]
        n73 = property class="Clust"(reference=w172, error in=w171) -> (error out=w170:errorcluster, "Value"=w169:variant)  [unwired: 1 out]
        n74 = call "Gui_SetupVoltages.vi"("error in (no error)"=w170, "Variant"=w169) -> ("error out"=w180:errorcluster, "Variant Output"=w168:variant)  [unwired: 8 in]
        n75 = property class="Clust"(reference=w172, error in=w180, "Value"=w168) -> (error out=w166:errorcluster)  [unwired: 1 out]
        n76 = call "UI_Update_Status.vi"("error in (no error)"=w166, "UI Status"=QMH_UI_Command."Waiting for User", "QMH UI Cluster"=w164) -> ("error out"=w165:errorcluster)  [unwired: 6 in, 2 out]
      }
      frame "UI Change Sequence" {
        n77 = call "UI_Update_Status.vi"("error in (no error)"=w197, "UI Status"=w198, "QMH UI Cluster"=w199) -> ("error out"=w201:errorcluster, "Variant"=w200:variant, "QMH UI Cluster"=w182:T35)  [unwired: 6 in]
        n78 = Unbundle By Name(w182) -> ("QMH UI References.Refnum EXPERT"=w192:refnum<vi>, "QMH UI References.Refnum SEQUENCE"=w195:refnum<vi>, "QMH UI References.Refnum EXCIT Table"=w185:refnum<vi>)
        n79 = call "QMH_UI_Control_EnQueue.vi"("error in (no error)"=w201, "Variant"=w200, "Command"=QMH_UI_Command."Update Report", "UI Queue"=w196) -> ("error out"=w190:errorcluster)  [unwired: 6 in, 1 out]
        n80 = property class="Clust"(reference=w192) -> ("Value"=w191:variant)  [unwired: 1 in, 2 out]
        n81 = property class="Clust"(reference=w195) -> ("Value"=w194:variant)  [unwired: 1 in, 2 out]
        n82 = property class="Clust"(reference=w185, error in=w190) -> (error out=w189:errorcluster, "Value"=w188:variant)  [unwired: 1 out]
        n83 = call "Gui_SetupSequence.vi"("Variant For Path"=w191, "error in (no error)"=w189, "Excit Table Variant"=w188, "Variant"=w194) -> ("error out"=w203:errorcluster, "Excit Table Variant Output"=w184:variant, "Variant Output"=w193:variant)  [unwired: 5 in]
        n84 = property class="Clust"(reference=w195, error in=w203, "Value"=w193) -> (error out=w187:errorcluster)  [unwired: 1 out]
        n85 = property class="Clust"(reference=w185, error in=w187, "Value"=w184) -> (error out=w186:errorcluster)  [unwired: 1 out]
        n86 = call "UI_Update_Status.vi"("error in (no error)"=w186, "UI Status"=QMH_UI_Command."Waiting for User", "QMH UI Cluster"=w182) -> ("error out"=w183:errorcluster)  [unwired: 6 in, 2 out]
      }
      frame "UI Change Expert" {
        n87 = call "UI_Update_Status.vi"("error in (no error)"=w209, "UI Status"=w210, "QMH UI Cluster"=w204) -> ("error out"=w211:errorcluster)  [unwired: 6 in, 2 out]
        n88 = Unbundle By Name(w204) -> ("QMH UI References.Refnum EXPERT"=w208:refnum<vi>)
        n89 = call "Gui_SetupExpert.vi"("error in (no error)"=w211, "QMH UI References.Refnum EXPERT"=w208) -> ("error out"=w206:errorcluster)  [unwired: 9 in]
        n90 = call "UI_Update_Status.vi"("error in (no error)"=w206, "UI Status"=QMH_UI_Command."Waiting for User", "QMH UI Cluster"=w204) -> ("error out"=w205:errorcluster)  [unwired: 6 in, 2 out]
      }
      frame "UI Change Loops" {
        n91 = call "UI_Update_Status.vi"("error in (no error)"=w226, "UI Status"=w227, "QMH UI Cluster"=w224) -> ("error out"=w223:errorcluster, "Variant"=w220:variant, "QMH UI Cluster"=w212:T35)  [unwired: 6 in]
        n92 = Unbundle By Name(w212) -> ("QMH UI References.Refnum LOOPS"=w213:refnum<vi>)
        n93 = call "QMH_UI_Control_EnQueue.vi"("error in (no error)"=w223, "Variant"=w220, "Command"=QMH_UI_Command."Update Report", "UI Queue"=w222) -> ("error out"=w217:errorcluster)  [unwired: 6 in, 1 out]
        n94 = property class="Clust"(reference=w213, error in=w217) -> (error out=w216:errorcluster, "Value"=w219:variant)  [unwired: 1 out]
        n95 = call "Gui_SetupLoops.vi"("error in (no error)"=w216, "Variant"=w219) -> ("error out"=w215:errorcluster, "Variant Output"=w218:variant)  [unwired: 8 in]
        n96 = property class="Clust"(reference=w213, error in=w215, "Value"=w218) -> (error out=w214:errorcluster)  [unwired: 1 out]
        n97 = call "UI_Update_Status.vi"("error in (no error)"=w214, "UI Status"=QMH_UI_Command."Waiting for User", "QMH UI Cluster"=w212) -> ("error out"=w225:errorcluster)  [unwired: 6 in, 2 out]
      }
      frame "UI Change Scientist" {
        n98 = call "UI_Update_Status.vi"("error in (no error)"=w239, "UI Status"=w238, "QMH UI Cluster"=w235) -> ("error out"=w232:errorcluster, "Variant"=w230:variant, "QMH UI Cluster"=w229:T35)  [unwired: 6 in]
        n99 = call "QMH_UI_Control_EnQueue.vi"("error in (no error)"=w232, "Variant"=w230, "Command"=QMH_UI_Command."Update Report", "UI Queue"=w233) -> ("error out"=w231:errorcluster)  [unwired: 6 in, 1 out]
        n100 = call "UI_Update_Status.vi"("error in (no error)"=w231, "UI Status"=QMH_UI_Command."Waiting for User", "QMH UI Cluster"=w229) -> ("error out"=w237:errorcluster)  [unwired: 6 in, 2 out]
      }
      frame "UI Exit" {
        # "Generate the user event \"User Stop\" to stop the Loop of UI Events"
        n101 = call "QMH_ICR_Control_EnQueue.vi"("error in (no error)"=w244, "Command"=QMH_ICR_Command."Exit", "ICR Queue"=w241) -> ("error out"=w243:errorcluster)  [unwired: 7 in, 1 out]
        n102 = Release Queue(queue=w242, error in (no error)=w243) -> (error out=w250:errorcluster)  [unwired: 1 in, 2 out]
        n103 = Generate User Event(user event=w248, event data cluster=TRUE ("données d'événement")) -> (error out=w247:errorcluster)  [unwired: 2 in, 1 out]
        n104 = Merge Errors(w247, w250) -> (w246:errorcluster)
      }
      frame "Update Experiment" {
        n105 = Unbundle By Name(w266) -> ("QMH UI References.Refnum EXPERIMENT"=w261:refnum<vi>, "QMH UI References.Refnum LOOPS"=w265:refnum<vi>)
        n106 = Variant To Data(error in=w267, type=i16 0, Variant=w268) -> (data=w256:i16, error out=w264:errorcluster)
        n107 = property class="Clust"(reference=w261) -> ("Value"=w259:variant)  [unwired: 1 in, 2 out]
        n108 = property class="Clust"(reference=w265, error in=w264) -> (error out=w252:errorcluster, "Value"=w260:variant)  [unwired: 1 out]
        n109 = call "Gui_UpdateExperiment.vi"("Laser 3.Wavelength"=w256, "error in (no error)"=w252, "Variant Loops"=w260, "Variant Experiment"=w259) -> ("error out"=w262:errorcluster, "Variant Output"=w258:variant)  [unwired: 6 in]
        n110 = property class="Clust"(reference=w261, error in=w262, "Value"=w258) -> (error out=w263:errorcluster)  [unwired: 1 out]
        n111 = call "QMH_UI_Control_EnQueue.vi"("error in (no error)"=w263, "Command"=QMH_UI_Command."UI Save", "UI Queue"=w254) -> ("error out"=w255:errorcluster)  [unwired: 7 in, 1 out]
      }
      frame "Update Report" {
        w280 = T37 {"UI Status"=enum."Initialize", "ICR Status"=enum."Initialize", "QMH Status"=enum."Init"}  # QMH UI Report
        n112 = Variant To Data(error in=w276, type=w280, Variant=w281) -> (data=w273:T37, error out=w279:errorcluster)
        n113 = Bundle By Name(cluster=w271, "QMH UI Report"=w273) -> (w272:T35)
        n114 = Unbundle By Name(w273) -> ("UI Status"=w270:T38, "ICR Status"=w269:T39)  [unwired: 1 out]
        n115 = Unbundle By Name(w272) -> ("QMH UI References"=w274:T36)
        n116 = call "UI_Update_Controls.vi"("error in (no error)"=w279, "ICR Status"=w269, "UI Status"=w270, "QMH UI References"=w274) -> ("error out"=w275:errorcluster, "QMH UI References"=w278:T36)  [unwired: 6 in]
        n117 = Bundle By Name(cluster=w271, "QMH UI References"=w278) -> (w277:T35)
      }
      frame "Update ICR Status" {
        n118 = Variant To Data(error in=w294, type=QMH_ICR_Command."Initialize" ("Command"), Variant=w295) -> (data=w291:T39, error out=w287:errorcluster)
        n119 = Bundle By Name(cluster=w293, "QMH UI Report.ICR Status"=w291) -> (w284:T35)
        n120 = call "UI_Update_Status.vi"("error in (no error)"=w287, "UI Status"=QMH_UI_Command."Waiting for ICR", "QMH UI Cluster"=w284) -> ("error out"=w286:errorcluster, "Variant"=w283:variant, "QMH UI Cluster"=w285:T35)  [unwired: 6 in]
        n121 = call "QMH_UI_Control_EnQueue.vi"("error in (no error)"=w286, "Variant"=w283, "Command"=QMH_UI_Command."Update Report", "UI Queue"=w288) -> ("error out"=w289:errorcluster)  [unwired: 6 in, 1 out]
      }
      frame "Ready to Start" {
        n122 = call "UI_Update_Status.vi"("error in (no error)"=w299, "UI Status"=w300, "QMH UI Cluster"=w301) -> ("error out"=w303:errorcluster, "Variant"=w302:variant, "QMH UI Cluster"=w297:T35)  [unwired: 6 in]
        n123 = call "QMH_UI_Control_EnQueue.vi"("error in (no error)"=w303, "Variant"=w302, "Command"=QMH_UI_Command."Update Report", "UI Queue"=w298) -> ("error out"=w296:errorcluster)  [unwired: 6 in, 1 out]
      }
      frame "Waiting for ICR" {
        n124 = call "UI_Update_Status.vi"("error in (no error)"=w314, "UI Status"=w315, "QMH UI Cluster"=w316) -> ("error out"=w318:errorcluster, "Variant"=w317:variant, "QMH UI Cluster"=w305:T35)  [unwired: 6 in]
        n125 = To Variant(anything=w305) -> (Variant=w310:variant)
        n126 = call "QMH_UI_Control_EnQueue.vi"("error in (no error)"=w318, "Variant"=w317, "Command"=QMH_UI_Command."Update Report", "UI Queue"=w313) -> ("error out"=w309:errorcluster)  [unwired: 6 in, 1 out]
        n127 = call "QMH_ICR_Control_EnQueue.vi"("error in (no error)"=w309, "Variant"=w310, "Command"=QMH_ICR_Command."Sequence Loop Setup", "ICR Queue"=w311) -> ("error out"=w307:errorcluster)  [unwired: 6 in, 1 out]
        n128 = call "UI_Update_Status.vi"("error in (no error)"=w307, "UI Status"=QMH_UI_Command."Waiting for ICR", "QMH UI Cluster"=w305) -> ("error out"=w306:errorcluster)  [unwired: 6 in, 2 out]
      }
      frame Default {
        (unwired) errorcluster {"status"=FALSE, "code"=0, "source"=""} ("sortie d'erreur")
        # "La condition 'Par défaut' ne s'exécute que s'il y a un message qui n'est défini dans aucune des autres conditions.  Renvoyer une erreur."
        n129 = One Button Dialog(message="Invalid Message") -> ()  [unwired: 1 in, 1 out]
      }
    }
  }
  n130 = while "Producer Loop for UI events" {
    tunnel: w11 -> [w328]
    tunnel: [w322] -> w21
    shift-right: [w324] -> w20
    shift-left: w24 -> [w325]
    stop <- w329 stop-if-true
    # "Error : send a message Exit to\nthe top of the queue"
    n131 = event shown="[3] \"Change Sequence\": Value Change" {
      selector: w325 -> [_ _ _ _ _ _ _ _ _ _ _ _ _]
      dyn-events: [_ _ _ _ _ _ _ _ _ _ _ _ _] -> w324
      timeout: _ -> [_ _ _ _ _ _ _ _ _ _ _ _ _]
      tunnel: w328 -> [w332 w335 w338 w342 w346 w350 w354 w360 w364 w369 w373 w381 w383]
      tunnel: [w330 w336 w339 w343 w347 w351 w355 w358 w362 w368 w372 w380 _] -> w327
      tunnel: [w331 w337 w340 w344 w348 w352 w356 w359 w363 w367 w371 w381 w383] -> w326
      tunnel: [_ _ _ _ _ _ _ _ _ _ _ _ TRUE ("User Stop")] -> w323
      event "Load": Value Change {
        n132 = event-data() -> ()  [unwired: 2 out]
        n133 = call "QMH_UI_Control_EnQueue.vi"("Command"=QMH_UI_Command."UI Load", "UI Queue"=w332) -> ("error out"=w330:errorcluster, "UI Queue"=w331:refnum<queue>)  [unwired: 8 in]
      }
      event "Change Experiment": Value Change {
        n134 = event-data() -> ()  [unwired: 2 out]
        n135 = call "QMH_UI_Control_EnQueue.vi"("Command"=QMH_UI_Command."UI Change Experiment", "UI Queue"=w335) -> ("error out"=w336:errorcluster, "UI Queue"=w337:refnum<queue>)  [unwired: 8 in]
      }
      event "Change Voltages": Value Change {
        n136 = event-data() -> ()  [unwired: 2 out]
        n137 = call "QMH_UI_Control_EnQueue.vi"("Command"=QMH_UI_Command."UI Change Voltages", "UI Queue"=w338) -> ("error out"=w339:errorcluster, "UI Queue"=w340:refnum<queue>)  [unwired: 8 in]
      }
      event "Change Sequence": Value Change {
        n138 = event-data() -> ()  [unwired: 2 out]
        n139 = call "QMH_UI_Control_EnQueue.vi"("Command"=QMH_UI_Command."UI Change Sequence", "UI Queue"=w342) -> ("error out"=w343:errorcluster, "UI Queue"=w344:refnum<queue>)  [unwired: 8 in]
      }
      event "Change Expert": Value Change {
        n140 = event-data() -> ()  [unwired: 2 out]
        n141 = call "QMH_UI_Control_EnQueue.vi"("Command"=QMH_UI_Command."UI Change Expert", "UI Queue"=w346) -> ("error out"=w347:errorcluster, "UI Queue"=w348:refnum<queue>)  [unwired: 8 in]
      }
      event "Change Loops": Value Change {
        n142 = event-data() -> ()  [unwired: 2 out]
        n143 = call "QMH_UI_Control_EnQueue.vi"("Command"=QMH_UI_Command."UI Change Loops", "UI Queue"=w350) -> ("error out"=w351:errorcluster, "UI Queue"=w352:refnum<queue>)  [unwired: 8 in]
      }
      event "Change Scientist": Value Change {
        n144 = event-data() -> ()  [unwired: 2 out]
        n145 = call "QMH_UI_Control_EnQueue.vi"("Command"=QMH_UI_Command."UI Change Scientist", "UI Queue"=w354) -> ("error out"=w355:errorcluster, "UI Queue"=w356:refnum<queue>)  [unwired: 8 in]
      }
      event "Save As": Value Change {
        n146 = event-data() -> ()  [unwired: 2 out]
        n147 = call "QMH_UI_Control_EnQueue.vi"("Command"=QMH_UI_Command."UI Save As", "UI Queue"=w360) -> ("error out"=w358:errorcluster, "UI Queue"=w359:refnum<queue>)  [unwired: 8 in]
      }
      event "Start": Value Change {
        n148 = event-data() -> ()  [unwired: 2 out]
        n149 = call "QMH_UI_Control_EnQueue.vi"("Command"=QMH_UI_Command."UI Start", "UI Queue"=w364) -> ("error out"=w362:errorcluster, "UI Queue"=w363:refnum<queue>)  [unwired: 8 in]
      }
      event "Exit": Value Change {
        n150 = event-data() -> ()  [unwired: 2 out]
        n151 = call "QMH_UI_Control_EnQueue.vi"("Command"=QMH_UI_Command."UI Exit", "UI Queue"=w369) -> ("error out"=w368:errorcluster, "UI Queue"=w367:refnum<queue>)  [unwired: 8 in]
      }
      event Menu Selection (User) {
        n152 = event-data() -> ("ItemTag"=w370:string)  [unwired: 1 out]
        n153 = case shown="\"Exit\"" w370 {
          tunnel: w373 -> [w377 w378]
          tunnel: [w375 w379] -> w372
          tunnel: [w376 w378] -> w371
          frame "Exit" {
            n154 = call "QMH_UI_Control_EnQueue.vi"("Command"=QMH_UI_Command."UI Exit", "UI Queue"=w377) -> ("error out"=w375:errorcluster, "UI Queue"=w376:refnum<queue>)  [unwired: 8 in]
          }
          frame "About", Default {
            n155 = call "Gui_About.vi"() -> ("error out"=w379:errorcluster)  [unwired: 11 in]
          }
        }
      }
      event "Excit Test": Value Change {
        n156 = event-data() -> ()  [unwired: 2 out]
        n157 = call "Hard_AWG_5421_Standard_Function.vi"() -> ("error out"=w380:errorcluster)  [unwired: 11 in]
      }
      event User Event {
        n158 = event-data() -> ()  [unwired: 3 out]
      }
    }
    n159 = case shown="Error" w327 {
      selector: w327 -> [w384 _]
      tunnel: [w385 TRUE] -> w329
      tunnel: w326 -> [_ w389]
      tunnel: w323 -> [w385 _]
      tunnel: [w384 w386] -> w322
      frame No Error {
      }
      frame Error {
        n160 = call "QMH_UI_Control_EnQueue.vi"("Last ?"=FALSE, "Command"=QMH_UI_Command."UI Exit", "UI Queue"=w389) -> ("error out"=w386:errorcluster)  [unwired: 7 in, 1 out]
      }
    }
  }
  n161 = Unregister For Events(event registration refnum=w20, error in=w21) -> (error out=w17:errorcluster)
  n162 = Destroy User Event(user event=w18, error in=w17) -> (error out=w16:errorcluster)
  n163 = Merge Errors(w16, w19, w9) -> (w12:errorcluster)
  n164 = property on="Property Node" class="App"(error in=w12) -> (error out=w15:errorcluster, "App.Kind"=w14:T44)  [unwired: 1 in, 1 out]
  n165 = call <vilib>:"Simple Error Handler.vi"("error in (no error)"=w15) -> ("error out"=w13:errorcluster)  [unwired: 4 in, 4 out]
  n166 = case shown="\"Run Time System\"" w14 {
    tunnel: w13 -> [_ _]
    frame Default {
    }
    frame "Run Time System" {
      n167 = Quit LabVIEW() -> ()  [unwired: 1 in]
    }
  }
